vi "MouseDoubleClick Response.vi"(4 "PlatMods":T1, 6 "Mods":cluster{"Double Click":bool, "Menu Key":bool}, 8 "error in (no error)":errorcluster, 9 "Button":u16, 10 "Coords":T2, 11 "Editor Handler in":refnum<class "Image Editor Handler.lvclass">) -> (0 "error out":errorcluster, 3 "Editor Handler out":refnum<class "Image Editor Handler.lvclass">)   [LabVIEW 2015, in "LV Image Editor Framework.lvlib" / "Image Editor Handler.lvclass"]
uses:
  Image Editor Handler.lvclass
  <vilib>/Utility/miscctls.llb/LVPoint32TypeDef.ctl
  Image Editor Handler.lvclass/Image Editor Handler.ctl
  Forms/Shape/Shape.lvclass
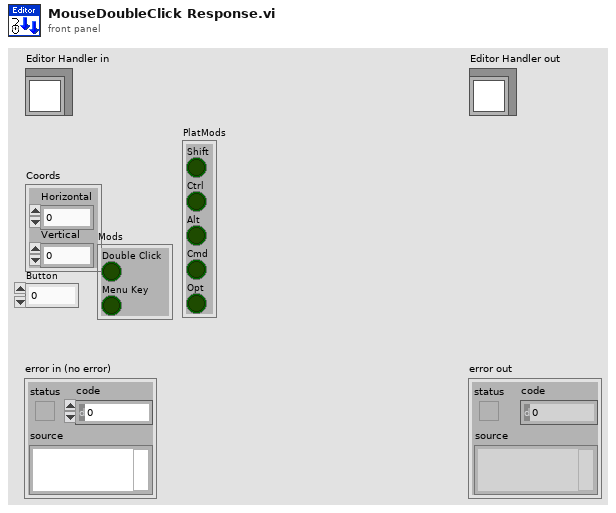
[diagram p1: front panel]
types:
  T1 = cluster{"Shift":bool, "Ctrl":bool, "Alt":bool, "Cmd":bool, "Opt":bool}
  T2 = typedef "LVPoint32TypeDef.ctl" = cluster{"Horizontal":i32, "Vertical":i32}
  T3 = typedef "LVPositionTypeDef.ctl" = cluster{"Left":i32, "Top":i32}
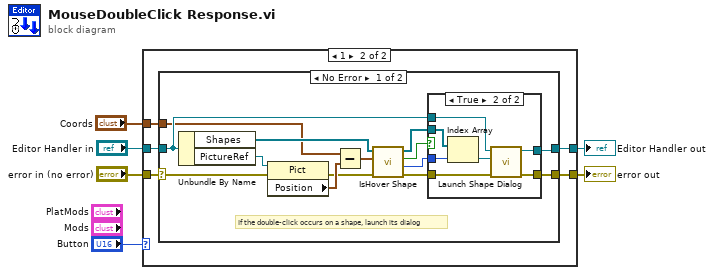
[diagram p0: block diagram]
diagram:
  n1 = case shown="1" "Button" {
    tunnel: "error in (no error)" -> [w7 w13]
    tunnel: [w7 w12] -> w5
    tunnel: "Editor Handler in" -> [w8 w11]
    tunnel: [w8 w10] -> w3
    tunnel: "Coords" -> [_ w9]
    frame 0, Default {
    }
    frame 1 {
      n2 = case shown="No Error" w13 {
        selector: w13 -> [w15 w38]
        tunnel: [w20 w38] -> w12
        tunnel: [w22 w37] -> w10
        tunnel: w11 -> [w23 w37]
        tunnel: w9 -> [w18 _]
        frame No Error {
          # "If the double-click occurs on a shape, launch its dialog"
          n3 = Unbundle By Name(w23) -> ("Shapes"=w27:refnum<data-value>[], "PictureRef"=w16:refnum<vi>)
          n4 = property class="Pict"(reference=w16, error in=w15) -> (error out=w14:errorcluster, "Position"=w19:T3)  [unwired: 1 out]
          n5 = Subtract(x=w18, y=w19) -> (x-y=w17:T2)
          n6 = call "IsHover Shape.vi"("error in (no error)"=w14, "Coords"=w17, "Shape in"=w27) -> ("error out"=w21:errorcluster, "Node ID"=w24:i32, "Found?"=w26:bool, "Shape out"=w25:refnum<data-value>[])  [unwired: 3 in, 2 out]
          n7 = case shown="True" w26 {
            tunnel: w25 -> [_ w36]
            tunnel: w24 -> [_ w35]
            tunnel: w23 -> [w29 w34]
            tunnel: [w29 w33] -> w22
            tunnel: w21 -> [w28 w32]
            tunnel: [w28 w31] -> w20
            frame False {
            }
            frame True {
              n8 = Index Array(array=w36, index=w35) -> (element=w30:refnum<data-value>)
              n9 = call "Launch Shape Dialog.vi"("error in (no error)"=w32, "ShapeRef"=w30, "Editor Handler in"=w34) -> ("error out"=w31:errorcluster, "Editor Handler out"=w33:refnum<class "Image Editor Handler.lvclass">)  [unwired: 7 in]
            }
          }
        }
        frame Error {
        }
      }
    }
  }
  "error out" <- w5
  "Editor Handler out" <- w3
